vi "PmacFileDownLoadLog.vi"(0 "Log File Path":path) -> ()   [LabVIEW 2020]
doc: "Load the down load compile log file generated by PmacFileDownLoad and display the contents. This panel automatically appears if an error occurs during the down load process. The modal panel must be closed before continuing."
panel:
  in  "Close":bool
  out "Down Load Log File":string=";Log created by PMAC Win32 Driver from file: D:\\LabView\\PmacView.lib\\PmacTest\\PmacTestPQM2.pmc\n;\n000001:                                  Compiling for PLCC: D:\\LabView\\PmacView.lib\\PmacTest\\PmacTestPQM2.PMA = D:\\LabView\\PmacView.lib\\PmacTest\\PmacTestPQM2.56K\n000002:                                  PLCC Compiling PMAC file: D:\\LabView\\PmacView.lib\\PmacTest\\PmacTestPQM2.pmc\n000003:                                  Success in Compiling to output file: D:\\LabView\\PmacView.lib\\PmacTest\\PmacTestPQM2.56K\n000004:                                  No PLCC(s) were compiled\n000005:                                  Downloading file: D:\\LabView\\PmacView.lib\\PmacTest\\PmacTestPQM2.56K\n000006:                                  Total Warnings: 0\n000007:                                  Total Errors: 0\n000008:                                  END.\n"
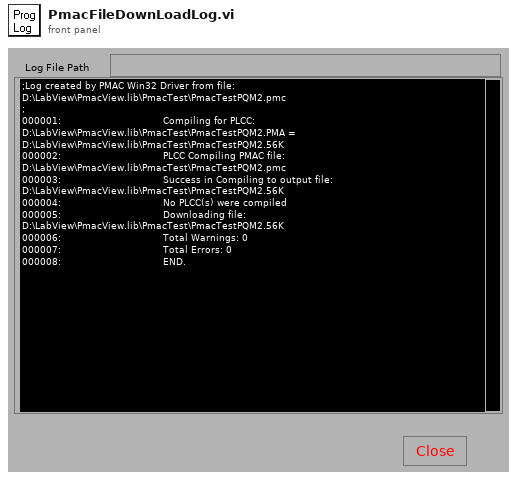
[diagram p1: front panel]
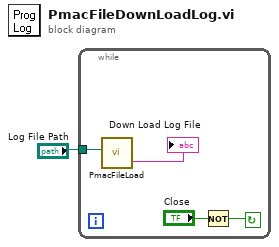
[diagram p0: block diagram]
diagram:
  n1 = while {
    tunnel: "Log File Path" -> [w2]
    stop <- w4 continue-if-true
    n2 = call "PmacFileLoad.vi"("Input Path (dialog if empty)"=w2) -> ("Buffer String"=→"Down Load Log File":string)  [unwired: 1 out]
    n3 = Not(x="Close") -> (.not. x?=w4:bool)
  }
